vi "SubVI_GetCamDevices.vi"(11 "ErrorIn":errorcluster) -> (0 "au32CameraSerials":u32[](array[numeric]), 1 "u32NumberOfCameras":u32, 3 "ErrorOut":errorcluster, 4 "strCameraDeviceType":cluster{string, "Output":u32}[](array[cluster]), 6 "u8Error":u8)   [LabVIEW 2013]
uses:
  <vilib>/Utility/importsl/GetValueByPointer/datatype.ctl
  <vilib>/Utility/importsl/GetValueByPointer/GetValueByPointer.xnode
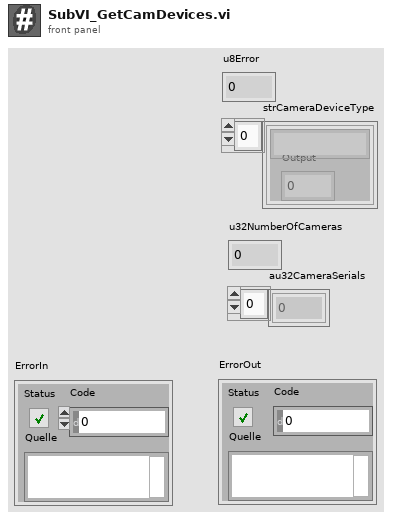
[diagram p1: front panel]
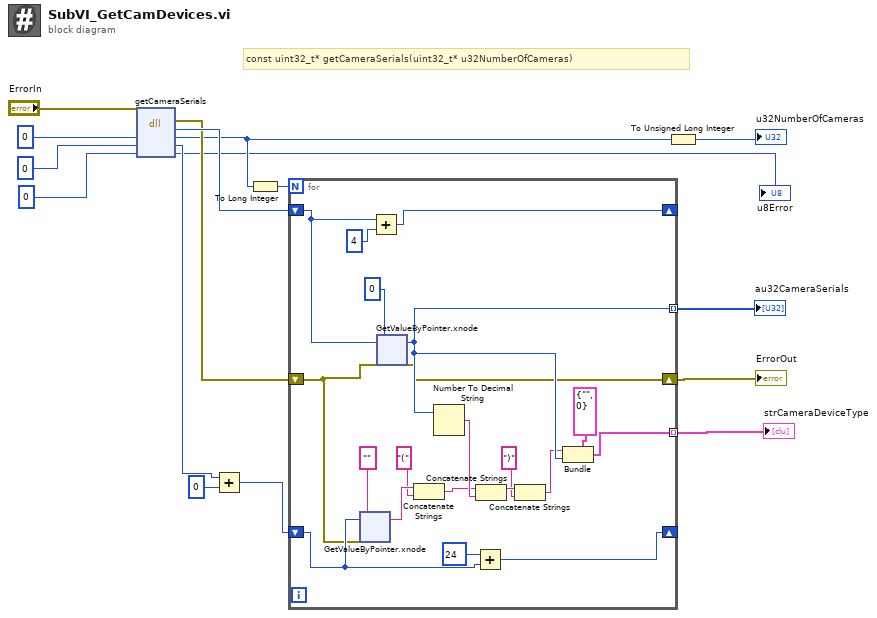
[diagram p0: block diagram]
diagram:
  # "const uint32_t* getCameraSerials(uint32_t* u32NumberOfCameras)"
  n1 = dll-call lib="PTH1abs CUsers1000len-bimDesktop&Lieferung_LabView_Interface_11.11.2015Einrichten fÃ¼r - EndkundenDatenTesto_v2013VIlabview_cwrapper_1_0_0.dll" fn="getCameraSerials"(error in="ErrorIn", "u32NumberOfCameras"=u64 0 ("u32NumberOfCameras*"), "psCurrentDeviceIds"=u64 0 ("arg1"), "u8Error"=u8 0) -> (error out=w10:errorcluster, "u32CameraSerials"=w14:u64, "u32NumberOfCameras"=w4:u64, "psCurrentDeviceIds"=w6:u64, "u8Error"=→"u8Error":u8)  [unwired: 2 in, 1 out]
  n2 = Add(x=w6, y=u64 0) -> (x+y=w8:u64)
  n3 = To Long Integer(number=w4) -> (32bit integer=w13:i32)
  n4 = for "For-Schleife" {
    N: w13 -> [_]
    shift-right: [w36] -> _
    shift-left: w14 -> [w31]
    tunnel: [w33] -> w16 mode=indexing
    tunnel: [w32] -> w15 mode=indexing
    shift-right: [w29] -> w9
    shift-left: w10 -> [w18]
    shift-right: [w27] -> _
    shift-left: w8 -> [w26]
    n5 = xnode "GetValueByPointer.xnode"("Pointer"=w26, "InputType"="", "ErrorIn"=w18) -> ("Output"=w24:string)  [unwired: 1 in, 1 out]
    n6 = Add(x=w31, y=u64 4) -> (x+y=w36:u64)
    n7 = xnode "GetValueByPointer.xnode"("Pointer"=w31, "InputType"=u32 0 ("y"), "ErrorIn"=w18) -> ("Output"=w33:u32, "ErrorOut"=w29:errorcluster)  [unwired: 1 in]
    n8 = Concatenate Strings(w24, "(" ("String")) -> (w22:string)
    n9 = Number To Decimal String(number=w33) -> (decimal integer string=w30:string)  [unwired: 1 in]
    n10 = Add(x=u64 24, y=w26) -> (x+y=w27:u64)
    n11 = Concatenate Strings(w22, w30) -> (w21:string)
    n12 = Concatenate Strings(w21, ")" ("String")) -> (w19:string)
    n13 = Bundle(cluster=cluster{"String":string, "Value":u32} {"String"="", "Value"=0}, "String"=w19, "Value"=w33) -> (w32:cluster{"String":string, "Value":u32})
  }
  "au32CameraSerials" <- w16
  "strCameraDeviceType" <- w15
  "ErrorOut" <- w9
  n14 = To Unsigned Long Integer(number=w4) -> (unsigned 32bit integer=→"u32NumberOfCameras":u32)
